vi "(Sub) LastRun Path.vi"() -> (16 "LastRun Path":path, 17 "Config Path":path)   [LabVIEW 2017]
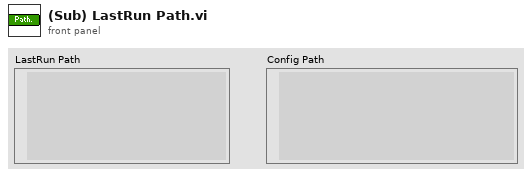
[diagram p1: front panel]
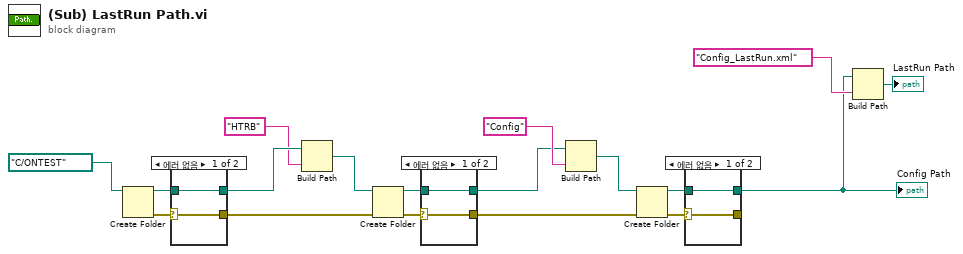
[diagram p0: block diagram]
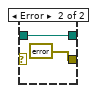
[diagram p2: hidden frame]
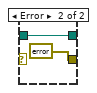
[diagram p3: hidden frame]
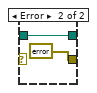
[diagram p4: hidden frame]
diagram:
  n1 = Create Folder(path (use dialog)=path "C:/ONTEST" ("path")) -> (created path=w16:path, error out=w17:errorcluster)  [unwired: 2 in, 1 out]
  n2 = case shown="에러 없음" w17 {
    selector: w17 -> [w20 _]
    tunnel: [w20 errorcluster {"status"=FALSE, "code"=0, "source"=""} ("에러 상수")] -> w10
    tunnel: w16 -> [w19 w21]
    tunnel: [w19 w21] -> w11
    frame No Error {
    }
    frame Error {
    }
  }
  n3 = Build Path(base path=w11, name or relative path="HTRB" ("이름 또는 상대 경로")) -> (appended path=w8:path)
  n4 = Create Folder(path (use dialog)=w8, error in=w10) -> (created path=w13:path, error out=w12:errorcluster)  [unwired: 1 in, 1 out]
  n5 = case shown="에러 없음" w12 {
    selector: w12 -> [w24 _]
    tunnel: [w24 errorcluster {"status"=FALSE, "code"=0, "source"=""} ("에러 상수")] -> w2
    tunnel: w13 -> [w23 w25]
    tunnel: [w23 w25] -> w3
    frame No Error {
    }
    frame Error {
    }
  }
  n6 = Build Path(base path=w3, name or relative path="Config" ("이름 또는 상대 경로")) -> (appended path=w7:path)
  n7 = Create Folder(path (use dialog)=w7, error in=w2) -> (created path=w4:path, error out=w5:errorcluster)  [unwired: 1 in, 1 out]
  n8 = case shown="에러 없음" w5 {
    selector: w5 -> [w28 _]
    tunnel: [w28 errorcluster {"status"=FALSE, "code"=0, "source"=""} ("에러 상수")] -> _
    tunnel: w4 -> [w27 w29]
    tunnel: [w27 w29] -> w1
    frame No Error {
    }
    frame Error {
    }
  }
  "Config Path" <- w1
  n9 = Build Path(base path=w1, name or relative path="Config_LastRun.xml" ("이름 또는 상대 경로")) -> (appended path=→"LastRun Path":path)
